vi "ElevatorSim_Update.vi"(10 "dT_Seconds":dbl=0.02, 11 "in ElevatorSim":T1 {"GearBox"."Jr_KgM2" format="%13.5p"; "GearBox"."L_H" format="%13.5p"; "GearBox"."Kt_NMPerAmp" format="%13.5p"; "GearBox"."KvINV_RadPerSecPerVolt" format="%13.5p"; "GearBox"."R_Ohms" format="%13.5p"; "GearBox"."FreeSpeed_RadPerSec" format="%13.5p"; "GearBox"."FreeCurrent_Amps" format="%13.5p"; "GearBox"."StallCurrent_Amps" format="%13.5p"; "GearBox"."StallTorque_NM" format="%13.5p"; "GearBox"."nominalVoltage_Volts" format="%13.5p"}) -> (0 "Error":bool, 3 "out ElevatorSim":T1 {"GearBox"."Jr_KgM2" format="%13.5p"; "GearBox"."L_H" format="%13.5p"; "GearBox"."Kt_NMPerAmp" format="%13.5p"; "GearBox"."KvINV_RadPerSecPerVolt" format="%13.5p"; "GearBox"."R_Ohms" format="%13.5p"; "GearBox"."FreeSpeed_RadPerSec" format="%13.5p"; "GearBox"."FreeCurrent_Amps" format="%13.5p"; "GearBox"."StallCurrent_Amps" format="%13.5p"; "GearBox"."StallTorque_NM" format="%13.5p"; "GearBox"."nominalVoltage_Volts" format="%13.5p"})   [LabVIEW 2019, in "Trajectory_Library.lvlib"]
doc: "Updates the simulation.\n \nInputs:\n - ElevatorSim -- Data cluster\n - dtSeconds -- The time between updates.\n\nOutputs:\n - OutElevatorSim -- Updated data cluster\n - Error -- If TRUE, an error occured."
uses:
  Trajectory_Library.lvlib
  ELEVATOR_SIM.ctl
  LINEAR_SYSTEM_SIM.ctl
  LINEAR_SYSTEM.ctl
  <vilib>/Analysis/Matrix/Datatypes/RealMatrix.ctl
  DCMOTOR.CTL
  <vilib>/Analysis/Matrix/NI_Matrix.lvlib
panel:
  # "<1, 1>"
  # "<States, 1>"
  # "<Outputs, 1>"
  # "<Inputs, 1>"
  # "<Outputs, 1>"
  # "<States,States>"
  # "<States,Inputs>"
  # "<Outputs,States>"
  # "<Outputs,Inputs>"
  # "<States, 1>"
  # "<Outputs, 1>"
  # "<Inputs, 1>"
  # "<Outputs, 1>"
  # "<States,States>"
  # "<States,Inputs>"
  # "<Outputs,States>"
  # "<Outputs,Inputs>"
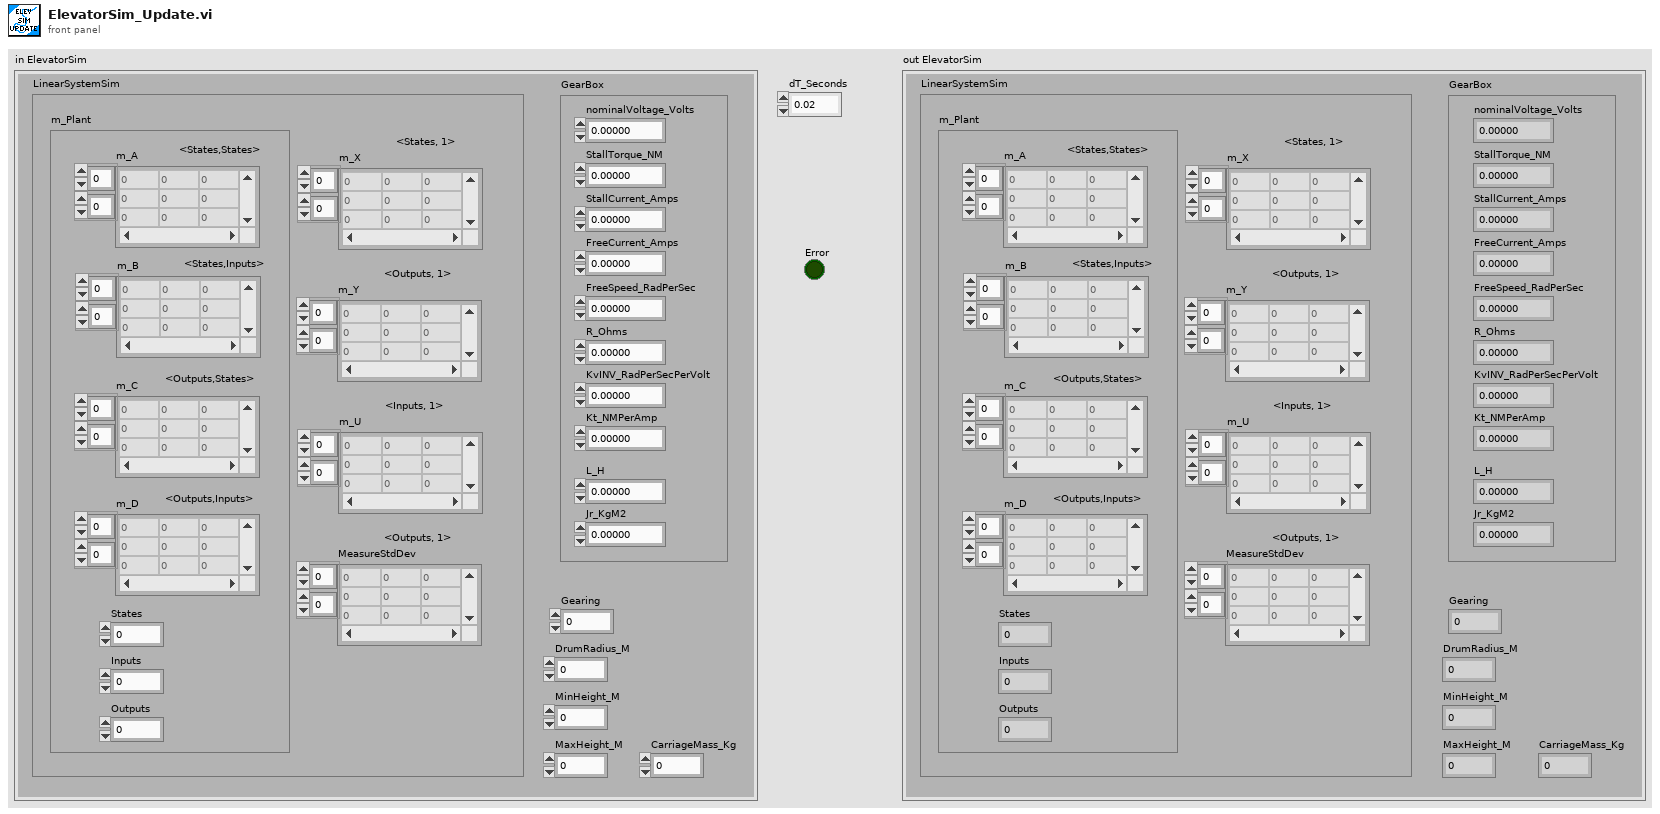
[diagram p1: front panel]
types:
  T1 = typedef "Trajectory_Library.lvlib/ELEVATOR_SIM.ctl" = cluster{"LinearSystemSim":T2, "GearBox":T5, "Gearing":dbl, "DrumRadius_M":dbl, "MinHeight_M":dbl, "MaxHeight_M":dbl, "CarriageMass_Kg":dbl}
  T2 = typedef "Trajectory_Library.lvlib/LINEAR_SYSTEM_SIM.ctl" = cluster{"m_Plant":T3, "m_X":T4, "m_Y":T4, "m_U":T4, "MeasureStdDev":T4}
  T3 = typedef "Trajectory_Library.lvlib/LINEAR_SYSTEM.ctl" = cluster{"m_A":T4, "m_B":T4, "m_C":T4, "m_D":T4, "States":i32, "Inputs":i32, "Outputs":i32}
  T4 = typedef "NI_Matrix.lvlib/RealMatrix.ctl" = dbl[][]
  T5 = typedef "Trajectory_Library.lvlib/DCMOTOR.CTL" = cluster{"nominalVoltage_Volts":dbl, "StallTorque_NM":dbl, "StallCurrent_Amps":dbl, "FreeCurrent_Amps":dbl, "FreeSpeed_RadPerSec":dbl, "R_Ohms":dbl, "KvINV_RadPerSecPerVolt":dbl, "Kt_NMPerAmp":dbl, "L_H":dbl, "Jr_KgM2":dbl}
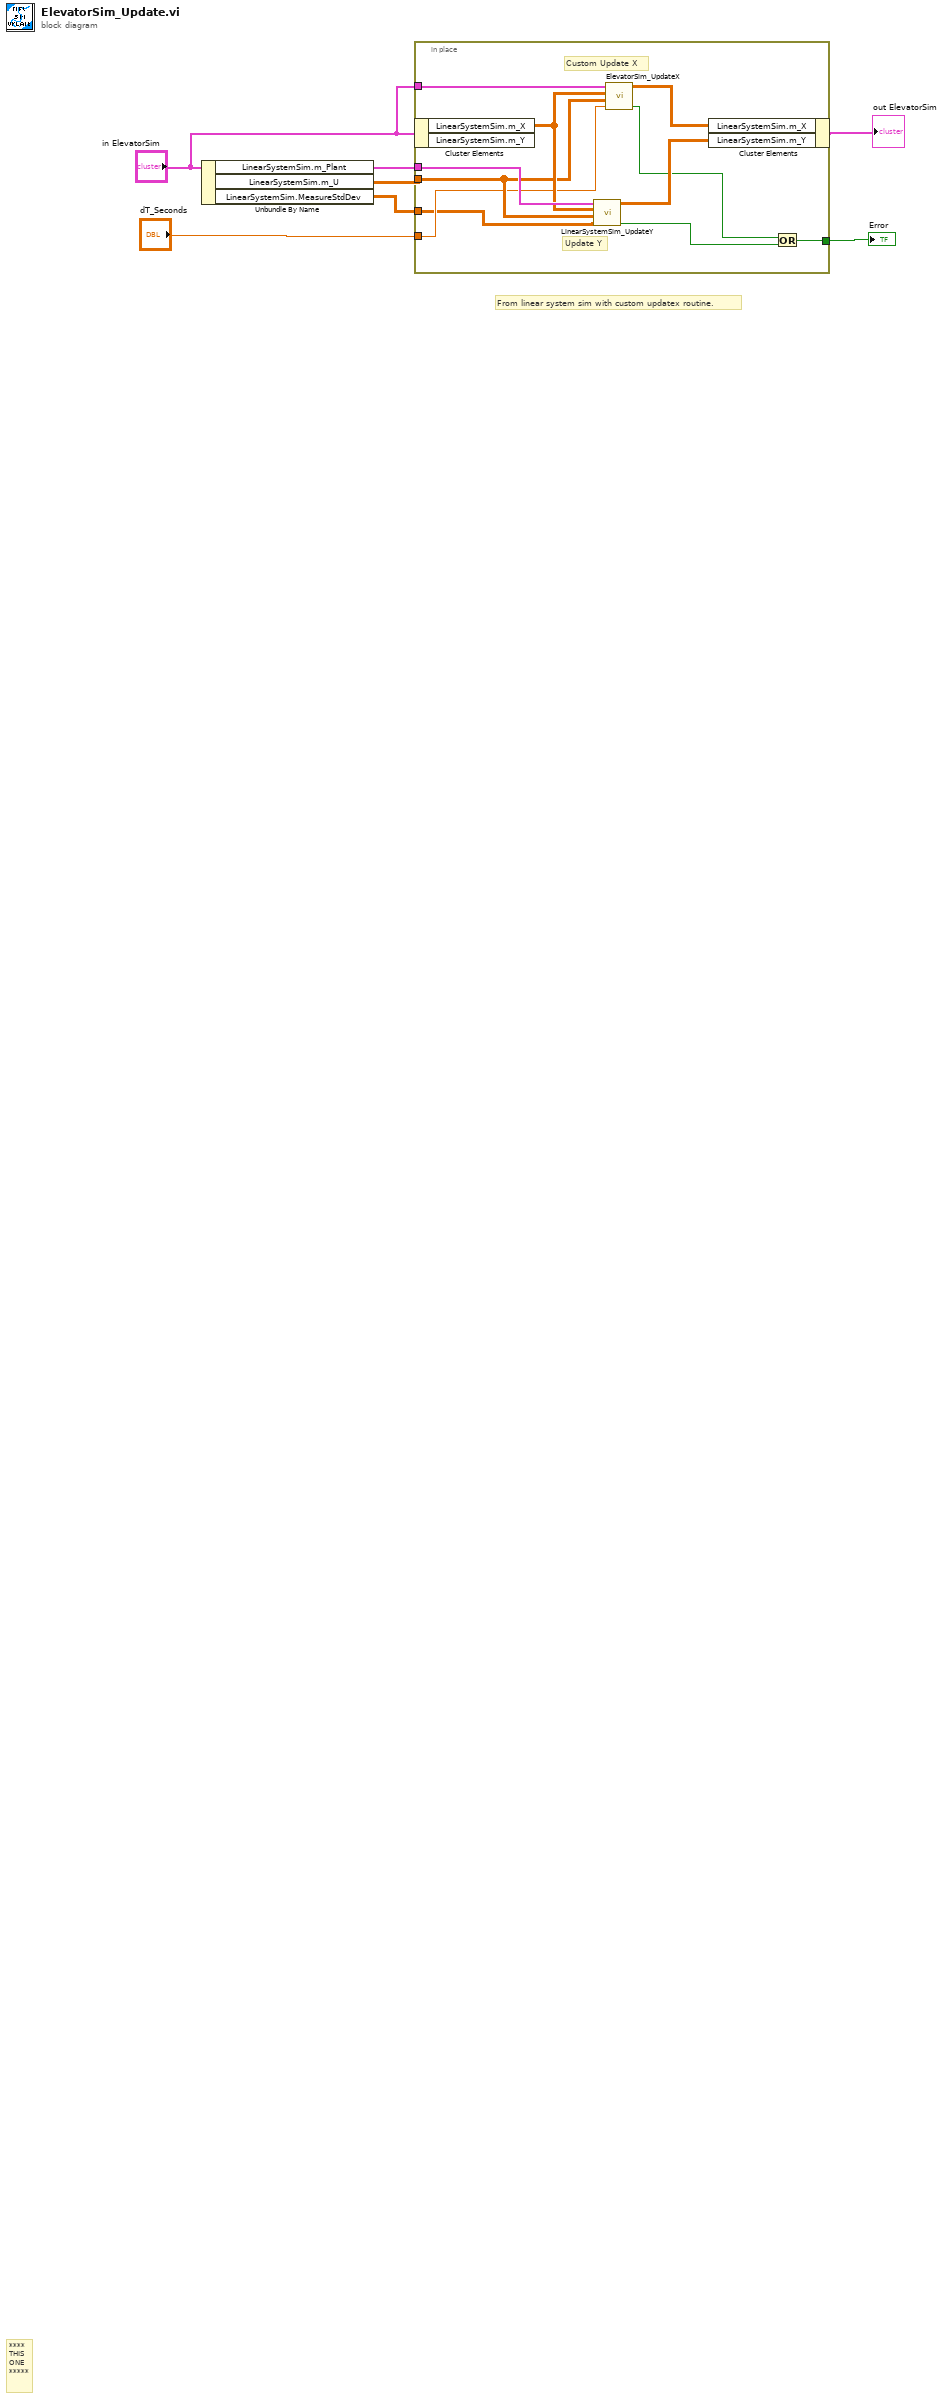
[diagram p0: block diagram]
diagram:
  # "From linear system sim with custom updatex routine."
  # "****\nTHIS\nONE\n*****"
  n1 = Unbundle By Name("in ElevatorSim") -> ("LinearSystemSim.m_Plant"=w4:T3, "LinearSystemSim.m_U"=w5:T4, "LinearSystemSim.MeasureStdDev"=w2:T4)
  n2 = in-place {
    in-place-border: w5 -> [w14]
    in-place-border: "dT_Seconds" -> [w13]
    in-place-border: "in ElevatorSim" -> [w12]
    in-place-border: w4 -> [w17]
    in-place-border: w2 -> [w11]
    in-place-border: [w10] -> w1
    # "Update Y"
    # "Custom Update X"
    n3 = in-place-cluster #1("in ElevatorSim") -> ("LinearSystemSim.m_X"=w15:T4)  [unwired: 1 out]
    n4 = call "LinearSystemSim_UpdateY.vi"("MeasurementStdDev"=w11, "ClampedU"=w14, "X"=w15, "Linearsystem"=w17) -> ("Error"=w8:bool, "Y"=w18:T4)  [unwired: 6 in]
    n5 = call "ElevatorSim_UpdateX.vi"("dT_Seconds"=w13, "U"=w14, "current_xHat"=w15, "ELEVATOR_SIM"=w12) -> ("Error"=w9:bool, "updated_xHat"=w16:T4)  [unwired: 6 in]
    n6 = in-place-cluster #1("LinearSystemSim.m_X"=w16, "LinearSystemSim.m_Y"=w18) -> (→"out ElevatorSim":T1)
    n7 = Or(x=w9, y=w8) -> (x .or. y?=w10:bool)
  }
  "Error" <- w1
